vi "GetExternalInterfaces.vi"(8 "ErrorIn":errorcluster, 11 "ReferenceIn":refnum<class "VerticalButtonBar.lvclass">) -> (0 "ErrorOut":errorcluster, 2 "ExternalInterfaces":T1[](array[typedef]), 3 "ReferenceIn":refnum<class "VerticalButtonBar.lvclass">)   [LabVIEW 2021, in "VerticalButtonBar.lvclass"]
doc: "Gets the external interface objects that are used by the object. Each interface is defined by:\n\n\n- the label of the control in the attribute cluster of the object\n\n- the object inself that inherits from the attribute control\n\n- a boolean that indicates if this an array of objects"
uses:
  VerticalButtonBar.lvclass
  Library_TAF_Support/ClusterArrayConversion/BundledArray.ctl
  c918bead-a22c-460a-a6f4-f95520c4e6a6.vi
  c918bead-a22c-460a-a6f4-f95520c4e6a6.vi/e733eca7-9823-4359-8665-3b184f9a7377.vi
  <vilib>/Utility/Data Type/Get Cluster Information.vi
  <vilib>/Utility/Data Type/Get Type Information.vi
  Library_TAF_Support/ClusterArrayConversion/ClusterArrayConversion.lvlib
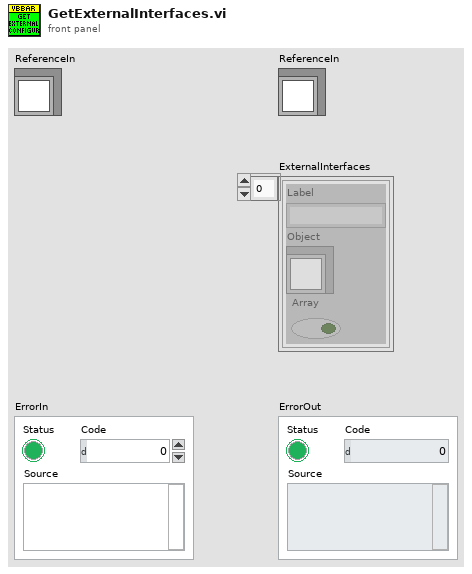
[diagram p1: front panel]
types:
  T1 = typedef "ClusterArrayConversion.lvlib/BundledArray.ctl" = cluster{"Label":string, "Object":refnum<class>, "Array":bool}
  T2 = typedef "VerticalButtonBar.lvclass/ObjectAttributes.ctl" = cluster{"Interfaces":cluster{"IDockGUI":refnum<class "IDockGUI.lvclass">, "Authorizer":refnum<class "IAuthorization.lvclass">}, "Locals":cluster{"ButtonBar":refnum<class "ButtonCollection.lvclass">, "BaseConfigurationPath":path, "Labels":cluster{"Label":string, "Value":string}[]}, "Persistent":cluster{"ButtonDefinitionFile":string}}
  T3 = cluster{"IDockGUI":refnum<class "IDockGUI.lvclass">, "Authorizer":refnum<class "IAuthorization.lvclass">}
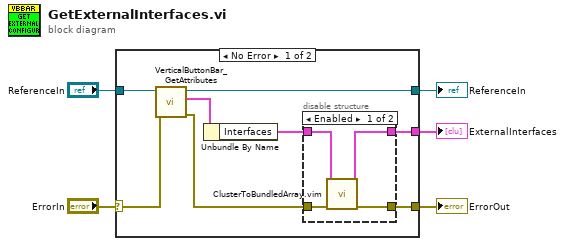
[diagram p0: block diagram]
diagram:
  n1 = case shown="No Error" "ErrorIn" {
    selector: "ErrorIn" -> [w13 w20]
    tunnel: [w11 w20] -> w4
    tunnel: [w8 w19] -> w2
    tunnel: "ReferenceIn" -> [w9 w19]
    tunnel: [w6 _] -> w1
    frame No Error {
      n2 = call "VerticalButtonBar_GetAttributes.vi"("ErrorIn"=w13, "ReferenceIn"=w9) -> ("ErrorOut"=w12:errorcluster, "Data"=w10:T2, "ReferenceOut"=w8:refnum<class "VerticalButtonBar.lvclass">)  [unwired: 6 in, 1 out]
      n3 = Unbundle By Name(w10) -> ("Interfaces"=w7:T3)
      n4 = disable-structure shown="Enabled" {
        disable-tunnel: w12 -> [w17 w18]
        disable-tunnel: w7 -> [w15 _]
        disable-tunnel: [w14 _] -> w6
        disable-tunnel: [w16 w18] -> w11
        frame Enabled {
          n5 = call "ClusterToBundledArray.vim"("ErrorIn"=w17, "Interfaces"=w15) -> ("ErrorOut"=w16:errorcluster, "BundeledLabels"=w14:T1[])  [unwired: 8 in]
        }
        frame Disabled {
        }
      }
    }
    frame Error {
    }
  }
  "ErrorOut" <- w4
  "ReferenceIn" <- w2
  "ExternalInterfaces" <- w1
